vi "BRig_RT__Case_Idle__State_Cue_pre.vi"(11 "input_dataMTrig":u16[](array[numeric])) -> (3 "output_dataMTrig":u16[](array[numeric]), 5 "output_state":T1)   [LabVIEW 2014]
uses:
  myRIO_BRig_RT__Case_NonExp_stateList.ctl
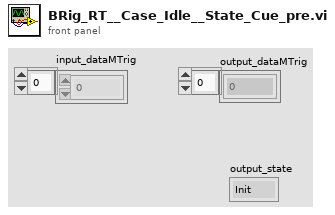
[diagram p1: front panel]
types:
  T1 = typedef "myRIO_BRig_RT__Case_NonExp_stateList.ctl" = enum16{"Init", "UploadSettings_pre", "UploadSettings_Read_dataExp", "UploadSettings_dataExp_1", "UploadSettings_dataExp_2", "UploadSettings_Read_dataLC", "UploadSettings_dataLC_1", "UploadSettings_dataLC_2", "UploadSettings_dataLC_3", "UploadSettings_dataLC_4", "UploadSettings_Read_dataMTrig", "UploadSettings_dataMTrig_1", "UploadSettings_post", "Idle_pre", "IdleEmpty", "IdleEmpty2", "IdleEmpty3", "IdleEmpty4", "Idle", "Idle_2", "Idle_3", "Idle_4", "Idle_5", "Idle_6", "Idle_post", "Cue_pre__pre", "Cue_pre", "Cue", "Cue_LED", "Cue_post", "RewardCalibration_pre", "RewardCalibration", "DispenseWater_pre__pre", "DispenseWater_pre", "DispenseWater", "DispenseWater_post", "TestConnection", "SendData", "Get_FPGA_count_per_ms", "End", "commTCP_connect"}
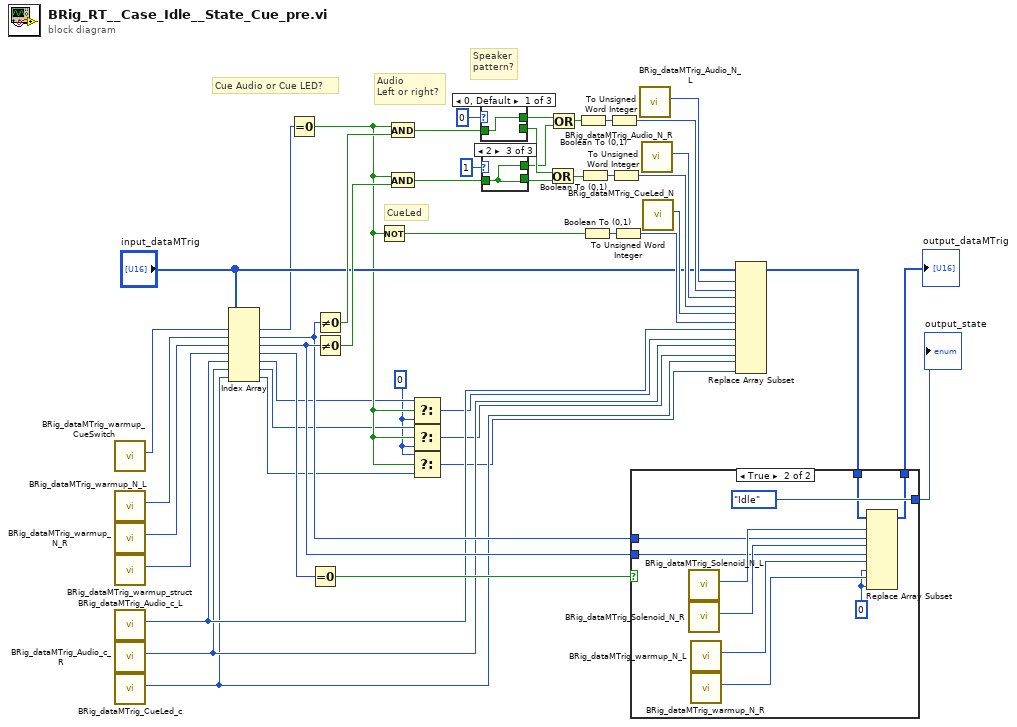
[diagram p0: block diagram]
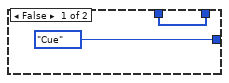
[diagram p2: hidden frame]
diagram:
  w7 = u16 0 ("f")
  # "Speaker\npattern?"
  # "CueLed"
  # "Audio\nLeft or right?"
  # "Cue Audio or Cue LED?"
  n1 = call "BRig_dataMTrig_warmup_CueSwitch.vi"() -> ("output_warmup_CueSwitch"=w13:i32)  [unwired: 11 in]
  n2 = call "BRig_dataMTrig_warmup_N_L.vi"() -> ("output_warmup_N_L"=w46:i32)  [unwired: 11 in]
  n3 = call "BRig_dataMTrig_warmup_N_R.vi"() -> ("output_warmup_N_R"=w45:i32)  [unwired: 11 in]
  n4 = call "BRig_dataMTrig_warmup_struct.vi"() -> ("output_warmup_struct"=w44:i32)  [unwired: 11 in]
  n5 = call "BRig_dataMTrig_Audio_c_L.vi"() -> ("output_Audio_c_L"=w6:i32)  [unwired: 11 in]
  n6 = call "BRig_dataMTrig_Audio_c_R.vi"() -> ("output_Audio_c_R"=w4:i32)  [unwired: 11 in]
  n7 = call "BRig_dataMTrig_CueLed_c.vi"() -> ("output_CueLed_c"=w2:i32)  [unwired: 11 in]
  n8 = Index Array(array="input_dataMTrig", index #1=w13, index #2=w46, index #3=w45, index #4=w44, index #5=w6, index #6=w4, index #7=w2) -> (element #1=w12:u16, element #2=w14:u16, element #3=w15:u16, element #4=w23:u16, element #5=w10:u16, element #6=w9:u16, element #7=w8:u16)
  n9 = Equal To 0?(x=w12) -> (x = 0?=w11:bool)
  n10 = Equal To 0?(x=w23) -> (x = 0?=w22:bool)
  n11 = Not Equal To 0?(x=w14) -> (x != 0?=w20:bool)
  n12 = Not Equal To 0?(x=w15) -> (x != 0?=w21:bool)
  n13 = Not(x=w11) -> (.not. x?=w39:bool)
  n14 = And(x=w11, y=w20) -> (x .and. y?=w42:bool)
  n15 = And(x=w11, y=w21) -> (x .and. y?=w40:bool)
  n16 = Select(t=w10, s=w11, f=w7) -> (s? t:f=w5:u16)
  n17 = Select(t=w9, s=w11, f=w7) -> (s? t:f=w3:u16)
  n18 = Select(t=w7, s=w11, f=w8) -> (s? t:f=w1:u16)
  n19 = case shown="0, Default" u16 0 {
    tunnel: [w47 _ w49] -> w34
    tunnel: [_ w48 w49] -> w35
    tunnel: w42 -> [w47 w48 w49]
    frame 0, Default {
    }
    frame 1 {
    }
    frame 2 {
    }
  }
  n20 = case shown="2" u16 1 ("sp_LeftSpout") {
    tunnel: [w50 _ w52] -> w33
    tunnel: [_ w51 w52] -> w36
    tunnel: w40 -> [w50 w51 w52]
    frame 0, Default {
    }
    frame 1 {
    }
    frame 2 {
    }
  }
  n21 = Or(x=w35, y=w36) -> (x .or. y?=w32:bool)
  n22 = Or(x=w34, y=w33) -> (x .or. y?=w30:bool)
  n23 = Boolean To (0,1)(Boolean=w30) -> (0, 1=w31:i16)
  n24 = Boolean To (0,1)(Boolean=w32) -> (0, 1=w37:i16)
  n25 = Boolean To (0,1)(Boolean=w39) -> (0, 1=w38:i16)
  n26 = To Unsigned Word Integer(number=w31) -> (unsigned 16bit integer=w26:u16)
  n27 = To Unsigned Word Integer(number=w37) -> (unsigned 16bit integer=w25:u16)
  n28 = To Unsigned Word Integer(number=w38) -> (unsigned 16bit integer=w24:u16)
  n29 = call "BRig_dataMTrig_Audio_N_L.vi"() -> ("output_Audio_N_L"=w29:i32)  [unwired: 11 in]
  n30 = call "BRig_dataMTrig_Audio_N_R.vi"() -> ("output_Audio_N_R"=w28:i32)  [unwired: 11 in]
  n31 = call "BRig_dataMTrig_CueLed_N.vi"() -> ("output_CueLed_N"=w27:i32)  [unwired: 11 in]
  n32 = Replace Array Subset(array="input_dataMTrig", new element #1=w26, index #1=w29, new element #2=w25, index #2=w28, new element #3=w24, index #3=w27, new element #4=w5, index #4=w6, new element #5=w3, index #5=w4, new element #6=w1, index #6=w2) -> (w19:u16[])
  n33 = case shown="True" w22 {
    tunnel: [myRIO_BRig_RT__Case_NonExp_stateList."Cue" ("Enum") myRIO_BRig_RT__Case_NonExp_stateList."Idle" ("Enum")] -> w16
    tunnel: w19 -> [w53 w63]
    tunnel: [w53 w62] -> w17
    tunnel: w15 -> [_ w56]
    tunnel: w14 -> [_ w55]
    frame False {
    }
    frame True {
      w57 = u16 0 ("new element/subarray")
      n34 = call "BRig_dataMTrig_Solenoid_N_L.vi"() -> ("output_Solenoid_N_L"=w61:i32)  [unwired: 11 in]
      n35 = call "BRig_dataMTrig_Solenoid_N_R.vi"() -> ("output_Solenoid_N_R"=w60:i32)  [unwired: 11 in]
      n36 = call "BRig_dataMTrig_warmup_N_L.vi"() -> ("output_warmup_N_L"=w59:i32)  [unwired: 11 in]
      n37 = call "BRig_dataMTrig_warmup_N_R.vi"() -> ("output_warmup_N_R"=w58:i32)  [unwired: 11 in]
      n38 = Replace Array Subset(array=w63, new element #1=w55, index #1=w61, new element #2=w56, index #2=w60, new element #3=w57, index #3=w59, new element #4=w57, index #4=w58) -> (w62:u16[])
    }
  }
  "output_dataMTrig" <- w17
  "output_state" <- w16
